vi "Read Measurement Counts.vi"(8 "error in (no error)":errorcluster, 11 "VISA resource name":refnum<visa-resource-name>) -> (0 "error out":errorcluster, 2 "Data Points":i32, 3 "VISA resource name out":refnum<visa-resource-name>)   [LabVIEW 2013, in "Agilent 3446X Series.lvlib"]
doc: "Returns the total number of measurements currently in reading memory."
uses:
  Agilent 3446X Series.lvlib
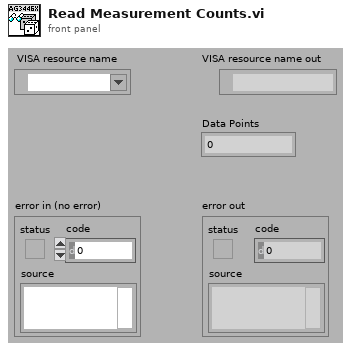
[diagram p1: front panel]
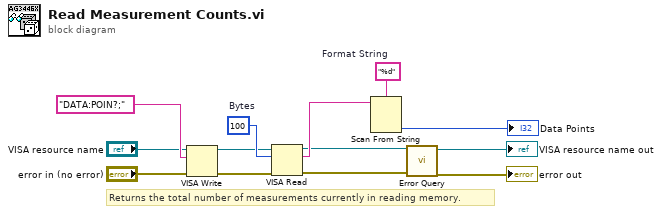
[diagram p0: block diagram]
diagram:
  w7 = "%d"  # Format String
  w8 = u32 100  # Bytes
  # "Returns the total number of measurements currently in reading memory."
  n1 = VISA Write(VISA resource name="VISA resource name", write buffer="DATA:POIN?;", error in (no error)="error in (no error)") -> (VISA resource name out=w5:refnum<visa-resource-name>, error out=w4:errorcluster)  [unwired: 1 out]
  n2 = VISA Read(VISA resource name=w5, byte count=w8, error in (no error)=w4) -> (VISA resource name out=w3:refnum<visa-resource-name>, read buffer=w6:string, error out=w2:errorcluster)  [unwired: 1 out]
  n3 = Scan From String(format string=w7, input string=w6) -> (output 1=→"Data Points":i32)  [unwired: 2 in, 4 out]
  n4 = call "Error Query.vi"("error in (no error)"=w2, "VISA resource name"=w3) -> ("error out"=→"error out":errorcluster, "VISA resource name out"=→"VISA resource name out":refnum<visa-resource-name>)  [unwired: 8 out]
